vi "ReadSSF_DSF.vi"(10 "DRWM path 2":path, 11 "DRWM path 1":path) -> (0 "DSF":cluster{"x":dbl, "y":dbl}[][](array[cluster]), 1 "因子棒号":string[](array[string]), 2 "SF_0K":bool, 3 "SSF":cluster{"x":dbl, "y":dbl}[][](array[cluster]), 5 "文件INFO":string)   [LabVIEW 2020]
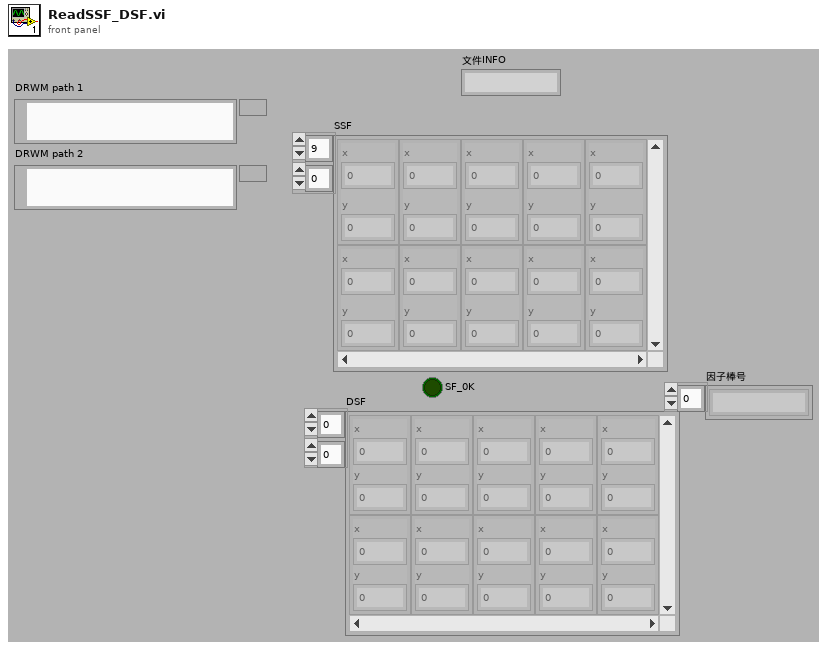
[diagram p1: front panel]
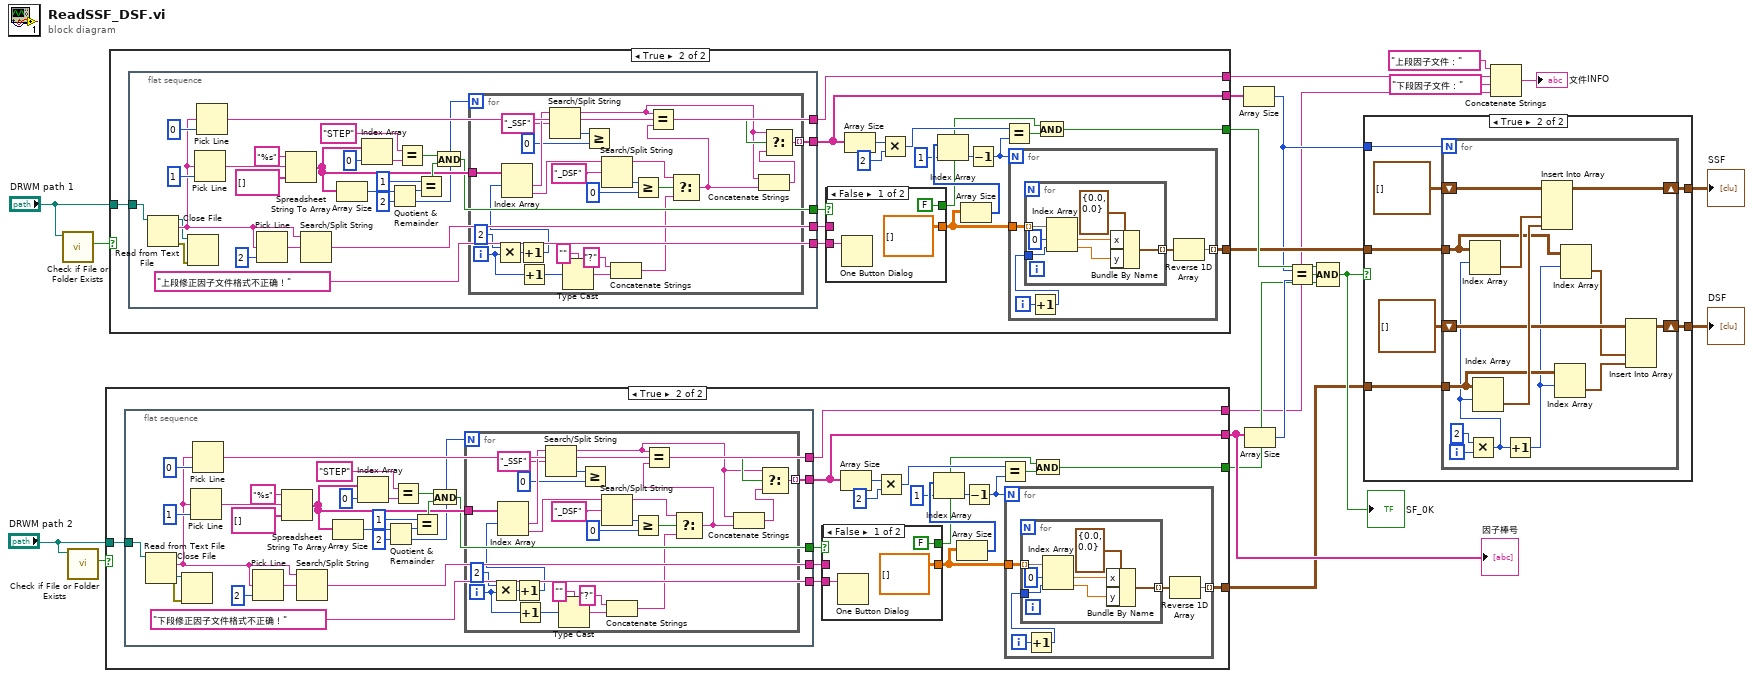
[diagram p0: block diagram]
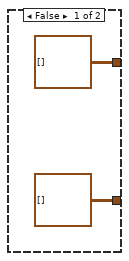
[diagram p2: hidden frame]
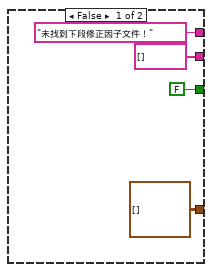
[diagram p3: hidden frame]
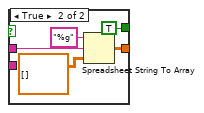
[diagram p4: hidden frame]
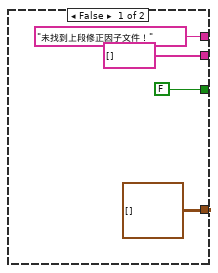
[diagram p5: hidden frame]
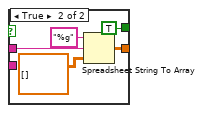
[diagram p6: hidden frame]
diagram:
  n1 = call <vilib>:"Check if File or Folder Exists.vi"("path"="DRWM path 1") -> ("file or folder exists?"=w21:bool)  [unwired: 8 in, 2 out]
  n2 = call <vilib>:"Check if File or Folder Exists.vi"("path"="DRWM path 2") -> ("file or folder exists?"=w20:bool)  [unwired: 8 in, 2 out]
  n3 = case shown="True" w20 {
    tunnel: [cluster{"x":dbl, "y":dbl}[][] [] w39] -> w12
    tunnel: "DRWM path 2" -> [_ w40]
    tunnel: [FALSE ("file or folder exists?") w28] -> w15
    tunnel: ["未找到下段修正因子文件！" ("output string") w27] -> w3
    tunnel: [string[] [] w26] -> w18
    frame False {
    }
    frame True {
      n4 = flat-sequence {
        tunnel: [w58] -> w43
        tunnel: [w77] -> w42
        tunnel: ["下段修正因子文件格式不正确！" ("消息")] -> w41
        tunnel: w40 -> [w59]
        tunnel: [w76] -> w27
        tunnel: [w61] -> w26
        frame #0 {
          n5 = Read from Text File(file (use dialog)=w59) -> (refnum out=w56:refnum<file>, text=w60:string, error out=w57:errorcluster)  [unwired: 3 in, 1 out]
          n6 = Close File(refnum=w56, error in=w57) -> ()  [unwired: 2 out]
          n7 = Pick Line ("选行并添加至字符串")(multi-line string=w60, line index=1 ("行索引")) -> (output string=w74:string)  [unwired: 1 in]
          n8 = Pick Line ("选行并添加至字符串")(multi-line string=w60, line index=0 ("行索引")) -> (output string=w76:string)  [unwired: 1 in]
          n9 = Pick Line ("选行并添加至字符串")(multi-line string=w60, line index=2 ("行索引")) -> (output string=w78:string)  [unwired: 1 in]
          n10 = Spreadsheet String To Array ("电子表格字符串至数组转换")(format string="%s" ("format (%.3f)"), spreadsheet string=w74, array type (2D Dbl)=string[] [] ("添加的数组")) -> (array=w63:string[])  [unwired: 1 in]
          n11 = Search/Split String(string=w60, search string/char (-)=w78) -> (match + rest of string=w77:string)  [unwired: 1 in, 2 out]
          n12 = Array Size(array=w63) -> (size(s)=w69:i32)
          n13 = Index Array(array=w63, index=0 ("索引")) -> (element=w71:string)
          n14 = Quotient & Remainder(x=w69, y=2) -> (x-y*floor(x/y)=w67:i32, floor(x/y)=w62:i32)
          n15 = Equal?(x="STEP", y=w71) -> (x = y?=w64:bool)
          n16 = Equal?(x=1, y=w67) -> (x = y?=w65:bool)
          n17 = And(x=w64, y=w65) -> (x .and. y?=w58:bool)
          n18 = for {
            N: w62 -> [_]
            tunnel: w63 -> [w107]
            tunnel: [w91] -> w61 mode=indexing
            i -> [w93]
            n19 = Multiply(x=2, y=w93) -> (x*y=w105:i32)
            n20 = Increment(x=w105) -> (x+1=w104:i32)
            n21 = Index Array(array=w107, index #1=w104) -> (element #1=w103:string, element #2=w96:string)  [unwired: 1 in]
            n22 = Increment(x=w93) -> (x+1=w92:i32)
            n23 = Search/Split String(string=w103, search string/char (-)="_SSF" ("搜索字符串/字符(-)")) -> (substring before match=w86:string, offset of match=w101:i32)  [unwired: 1 in, 1 out]
            n24 = Type Cast(type="" ("类型"), x=w92) -> (*(type *) &x=w90:string)
            n25 = Greater Or Equal?(x=w101, y=0) -> ()  [unwired: 1 out]
            n26 = Search/Split String(string=w96, search string/char (-)="_DSF" ("搜索字符串/字符(-)")) -> (substring before match=w88:string, offset of match=w98:i32)  [unwired: 1 in, 1 out]
            n27 = Concatenate Strings("?" ("字符串"), w90) -> (w85:string)
            n28 = Greater Or Equal?(x=w98, y=0) -> (x >= y?=w83:bool)
            n29 = Select(t=w88, s=w83, f=w85) -> (s? t:f=w84:string)
            n30 = Equal?(x=w86, y=w84) -> (x = y?=w95:bool)
            n31 = Concatenate Strings(w86, w84) -> (w87:string)
            n32 = Select(t=w86, s=w95, f=w87) -> (s? t:f=w91:string)
          }
        }
      }
      n33 = case shown="False" w43 {
        tunnel: w42 -> [_ w112]
        tunnel: [dbl[][] [] ("type (empty)") w113] -> w38
        tunnel: w41 -> [w109 _]
        tunnel: [FALSE ("file or folder exists?") TRUE ("file or folder exists?")] -> w29
        frame False {
          n34 = One Button Dialog(message=w109) -> ()  [unwired: 1 in, 1 out]
        }
        frame True {
          n35 = Spreadsheet String To Array ("电子表格字符串至数组转换")(format string="%g" ("format (%.3f)"), spreadsheet string=w112, array type (2D Dbl)=dbl[][] [] ("type (empty)")) -> (array=w113:dbl[][])  [unwired: 1 in]
        }
      }
      n36 = Array Size(array=w26) -> (size(s)=w34:i32)
      n37 = Multiply(x=w34, y=2) -> (x*y=w32:i32)
      n38 = Array Size(array=w38) -> (size(s)=w37:i32[])
      n39 = Index Array(array=w37, index=1 ("索引")) -> (element=w35:i32)
      n40 = Decrement(x=w35) -> (x-1=w31:i32)
      n41 = Equal?(x=w32, y=w31) -> (x = y?=w30:bool)
      n42 = for {
        N: w31 -> [_]
        tunnel: w38 -> [w47]
        tunnel: [w46] -> w39 mode=indexing
        i -> [w44]
        n43 = Increment(x=w44) -> (x+1=w45:i32)
        n44 = for {
          tunnel: w47 -> [w55] mode=indexing
          tunnel: [w53] -> w48 mode=indexing
          tunnel: w45 -> [w49]
          n45 = Index Array(array=w55, index #1=0 ("索引"), index #2=w49) -> (element #1=w51:dbl, element #2=w54:dbl)
          n46 = Bundle By Name(cluster=cluster{"x":dbl, "y":dbl} {"x"=0.0, "y"=0.0} ("输入簇"), "x"=w51, "y"=w54) -> (w53:cluster{"x":dbl, "y":dbl})
        }
        n47 = Reverse 1D Array(array=w48) -> (reversed array=w46:cluster{"x":dbl, "y":dbl}[])
      }
      n48 = And(x=w29, y=w30) -> (x .and. y?=w28:bool)
    }
  }
  "因子棒号" <- w18
  n49 = case shown="True" w21 {
    tunnel: [cluster{"x":dbl, "y":dbl}[][] [] w133] -> w13
    tunnel: "DRWM path 1" -> [_ w134]
    tunnel: [FALSE ("file or folder exists?") w122] -> w16
    tunnel: ["未找到上段修正因子文件！" ("output string") w121] -> w6
    tunnel: [string[] [] w120] -> w19
    frame False {
    }
    frame True {
      n50 = flat-sequence {
        tunnel: [w154] -> w137
        tunnel: [w171] -> w136
        tunnel: ["上段修正因子文件格式不正确！" ("消息")] -> w135
        tunnel: w134 -> [w152]
        tunnel: [w170] -> w121
        tunnel: [w155] -> w120
        frame #0 {
          n51 = Read from Text File(file (use dialog)=w152) -> (refnum out=w150:refnum<file>, text=w153:string, error out=w151:errorcluster)  [unwired: 3 in, 1 out]
          n52 = Close File(refnum=w150, error in=w151) -> ()  [unwired: 2 out]
          n53 = Pick Line ("选行并添加至字符串")(multi-line string=w153, line index=1 ("行索引")) -> (output string=w168:string)  [unwired: 1 in]
          n54 = Pick Line ("选行并添加至字符串")(multi-line string=w153, line index=0 ("行索引")) -> (output string=w170:string)  [unwired: 1 in]
          n55 = Pick Line ("选行并添加至字符串")(multi-line string=w153, line index=2 ("行索引")) -> (output string=w172:string)  [unwired: 1 in]
          n56 = Spreadsheet String To Array ("电子表格字符串至数组转换")(format string="%s" ("format (%.3f)"), spreadsheet string=w168, array type (2D Dbl)=string[] [] ("添加的数组")) -> (array=w157:string[])  [unwired: 1 in]
          n57 = Search/Split String(string=w153, search string/char (-)=w172) -> (match + rest of string=w171:string)  [unwired: 1 in, 2 out]
          n58 = Array Size(array=w157) -> (size(s)=w163:i32)
          n59 = Index Array(array=w157, index=0 ("索引")) -> (element=w165:string)
          n60 = Quotient & Remainder(x=w163, y=2) -> (x-y*floor(x/y)=w161:i32, floor(x/y)=w156:i32)
          n61 = Equal?(x="STEP", y=w165) -> (x = y?=w158:bool)
          n62 = Equal?(x=1, y=w161) -> (x = y?=w159:bool)
          n63 = And(x=w158, y=w159) -> (x .and. y?=w154:bool)
          n64 = for {
            N: w156 -> [_]
            tunnel: w157 -> [w201]
            tunnel: [w185] -> w155 mode=indexing
            i -> [w187]
            n65 = Multiply(x=2, y=w187) -> (x*y=w199:i32)
            n66 = Increment(x=w199) -> (x+1=w198:i32)
            n67 = Index Array(array=w201, index #1=w198) -> (element #1=w197:string, element #2=w190:string)  [unwired: 1 in]
            n68 = Increment(x=w187) -> (x+1=w186:i32)
            n69 = Search/Split String(string=w197, search string/char (-)="_SSF" ("搜索字符串/字符(-)")) -> (substring before match=w180:string, offset of match=w195:i32)  [unwired: 1 in, 1 out]
            n70 = Type Cast(type="" ("类型"), x=w186) -> (*(type *) &x=w184:string)
            n71 = Greater Or Equal?(x=w195, y=0) -> ()  [unwired: 1 out]
            n72 = Search/Split String(string=w190, search string/char (-)="_DSF" ("搜索字符串/字符(-)")) -> (substring before match=w182:string, offset of match=w192:i32)  [unwired: 1 in, 1 out]
            n73 = Concatenate Strings("?" ("字符串"), w184) -> (w179:string)
            n74 = Greater Or Equal?(x=w192, y=0) -> (x >= y?=w177:bool)
            n75 = Select(t=w182, s=w177, f=w179) -> (s? t:f=w178:string)
            n76 = Equal?(x=w180, y=w178) -> (x = y?=w189:bool)
            n77 = Concatenate Strings(w180, w178) -> (w181:string)
            n78 = Select(t=w180, s=w189, f=w181) -> (s? t:f=w185:string)
          }
        }
      }
      n79 = case shown="False" w137 {
        tunnel: w136 -> [_ w206]
        tunnel: [dbl[][] [] ("type (empty)") w207] -> w132
        tunnel: w135 -> [w203 _]
        tunnel: [FALSE ("file or folder exists?") TRUE ("file or folder exists?")] -> w123
        frame False {
          n80 = One Button Dialog(message=w203) -> ()  [unwired: 1 in, 1 out]
        }
        frame True {
          n81 = Spreadsheet String To Array ("电子表格字符串至数组转换")(format string="%g" ("format (%.3f)"), spreadsheet string=w206, array type (2D Dbl)=dbl[][] [] ("type (empty)")) -> (array=w207:dbl[][])  [unwired: 1 in]
        }
      }
      n82 = Array Size(array=w120) -> (size(s)=w128:i32)
      n83 = Multiply(x=w128, y=2) -> (x*y=w126:i32)
      n84 = Array Size(array=w132) -> (size(s)=w131:i32[])
      n85 = Index Array(array=w131, index=1 ("索引")) -> (element=w129:i32)
      n86 = Decrement(x=w129) -> (x-1=w125:i32)
      n87 = Equal?(x=w126, y=w125) -> (x = y?=w124:bool)
      n88 = for {
        N: w125 -> [_]
        tunnel: w132 -> [w141]
        tunnel: [w140] -> w133 mode=indexing
        i -> [w138]
        n89 = Increment(x=w138) -> (x+1=w139:i32)
        n90 = for {
          tunnel: w141 -> [w149] mode=indexing
          tunnel: [w147] -> w142 mode=indexing
          tunnel: w139 -> [w143]
          n91 = Index Array(array=w149, index #1=0 ("索引"), index #2=w143) -> (element #1=w145:dbl, element #2=w148:dbl)
          n92 = Bundle By Name(cluster=cluster{"x":dbl, "y":dbl} {"x"=0.0, "y"=0.0} ("输入簇"), "x"=w145, "y"=w148) -> (w147:cluster{"x":dbl, "y":dbl})
        }
        n93 = Reverse 1D Array(array=w142) -> (reversed array=w140:cluster{"x":dbl, "y":dbl}[])
      }
      n94 = And(x=w123, y=w124) -> (x .and. y?=w122:bool)
    }
  }
  n95 = Array Size(array=w19) -> (size(s)=w11:i32)
  n96 = Array Size(array=w18) -> (size(s)=w17:i32)
  n97 = Equal?(x=w11, y=w17) -> (x = y?=w10:bool)
  n98 = Compound Arithmetic op=AND(w16, w10, w15) -> (w14:bool)
  "SF_0K" <- w14
  n99 = case shown="True" w14 {
    tunnel: w13 -> [_ w217]
    tunnel: w12 -> [_ w216]
    tunnel: w11 -> [_ w218]
    tunnel: [cluster{"x":dbl, "y":dbl}[][] [] w214] -> w9
    tunnel: [cluster{"x":dbl, "y":dbl}[][] [] w212] -> w8
    frame False {
    }
    frame True {
      n100 = for {
        N: w218 -> [_]
        tunnel: w217 -> [w224]
        tunnel: w216 -> [w223]
        shift-right: [w229] -> w214
        shift-left: cluster{"x":dbl, "y":dbl}[][] [] -> [w230]
        shift-right: [w225] -> w212
        shift-left: cluster{"x":dbl, "y":dbl}[][] [] -> [w226]
        i -> [w232]
        n101 = Multiply(x=2, y=w232) -> (x*y=w222:i32)
        n102 = Index Array(array=w224, index (row)=w222) -> (element=w228:cluster{"x":dbl, "y":dbl}[])  [unwired: 1 in]
        n103 = Index Array(array=w223, index (row)=w222) -> (element=w227:cluster{"x":dbl, "y":dbl}[])  [unwired: 1 in]
        n104 = Increment(x=w222) -> (x+1=w221:i32)
        n105 = Insert Into Array(array=w230, new element #1=w228, new element #2=w227) -> (w229:cluster{"x":dbl, "y":dbl}[][])  [unwired: 2 in]
        n106 = Index Array(array=w223, index (row)=w221) -> (element=w219:cluster{"x":dbl, "y":dbl}[])  [unwired: 1 in]
        n107 = Index Array(array=w224, index (row)=w221) -> (element=w220:cluster{"x":dbl, "y":dbl}[])  [unwired: 1 in]
        n108 = Insert Into Array(array=w226, new element #1=w220, new element #2=w219) -> (w225:cluster{"x":dbl, "y":dbl}[][])  [unwired: 2 in]
      }
    }
  }
  "SSF" <- w9
  "DSF" <- w8
  n109 = Concatenate Strings("上段因子文件：" ("字符串"), w6, "下段因子文件：" ("字符串"), w3) -> (→"文件INFO":string)
